vi "Set Resource.vi"(8 "error in (no error)":errorcluster, 10 "Resource":T1, 11 "LangFile in":refnum<class "Resource Data.lvclass">) -> (0 "error out":errorcluster, 3 "LangFile out":refnum<class "Resource Data.lvclass">)   [LabVIEW 2013, in "SET Project Data.lvlib" / "Resource Data.lvclass"]
uses:
  Resource Data.lvclass
  Types/ProjFile_Resource Entry.ctl
  Resource Data.lvclass/Resource Data.ctl
  SET Project Data.lvlib
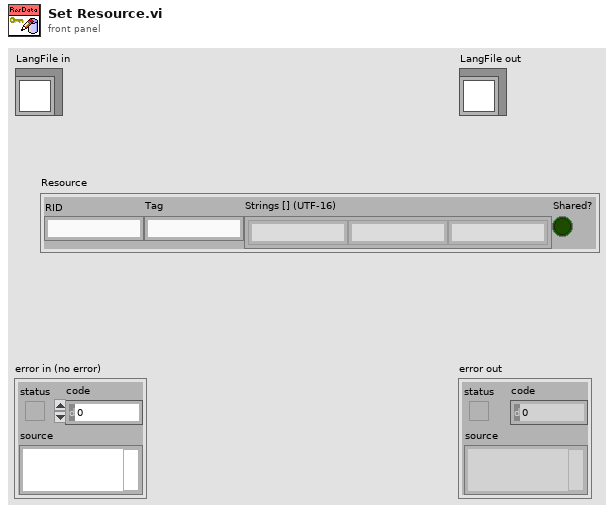
[diagram p1: front panel]
types:
  T1 = typedef "SET Project Data.lvlib/ProjFile_Resource Entry.ctl" = cluster{"RID":string, "Tag":string, "Strings [] (UTF-16)":string[], "Shared?":bool}
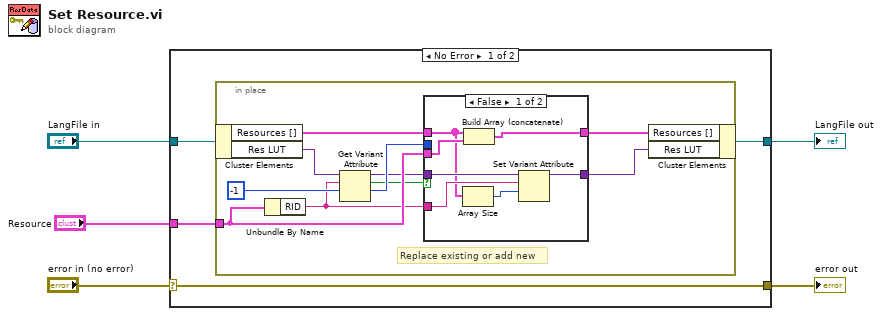
[diagram p0: block diagram]
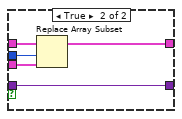
[diagram p2: hidden frame]
diagram:
  n1 = case shown="No Error" "error in (no error)" {
    selector: "error in (no error)" -> [w9 w33]
    tunnel: [w9 w33] -> w4
    tunnel: [w7 w32] -> w2
    tunnel: "LangFile in" -> [w8 w32]
    tunnel: "Resource" -> [w6 _]
    frame No Error {
      n2 = in-place {
        in-place-border: w6 -> [w14]
        # "Replace existing or add new"
        n3 = in-place-cluster #1(w8) -> ("Resources []"=w17:T1[], "Res LUT"=w19:variant)
        n4 = Unbundle By Name(w14) -> ("RID"=w11:string)
        n5 = Get Variant Attribute(Variant=w19, name=w11, default value (empty Variant)=-1) -> (duplicate Variant=w12:variant, found=w13:bool, value=w15:i32)  [unwired: 1 in, 1 out]
        n6 = case shown="False" w13 {
          tunnel: w17 -> [w23 w31]
          tunnel: [w20 w30] -> w16
          tunnel: w15 -> [_ w29]
          tunnel: w14 -> [w26 w28]
          tunnel: w12 -> [w25 w27]
          tunnel: w11 -> [w24 _]
          tunnel: [w21 w27] -> w10
          frame False {
            n7 = Array Size(array=w23) -> (size(s)=w22:i32)
            n8 = Build Array (concatenate)(w23, w26) -> (w20:T1[])
            n9 = Set Variant Attribute(Variant=w25, name=w24, value=w22) -> (Variant out=w21:variant)  [unwired: 1 in, 2 out]
          }
          frame True {
            n10 = Replace Array Subset(array=w31, new element=w28, index=w29) -> (w30:T1[])
          }
        }
        n11 = in-place-cluster #1("Resources []"=w16, "Res LUT"=w10) -> (w7:refnum<class "Resource Data.lvclass">)
      }
    }
    frame Error {
    }
  }
  "error out" <- w4
  "LangFile out" <- w2
